vi "ReceiveAsyncMessage.vi"(8 "error in (no error)":errorcluster, 11 "reference input":refnum<k24>) -> (0 "error out":errorcluster, 3 "reference output":refnum<k24>)   [LabVIEW 2013, in "main.lvlib"]
uses:
  main.lvlib
  C:/Users/Simon/SkyDrive/LabView/2013/DM2020/bin/medimatic_bt_receiver.dll
  bin/medimatic_bt_receiver.dll
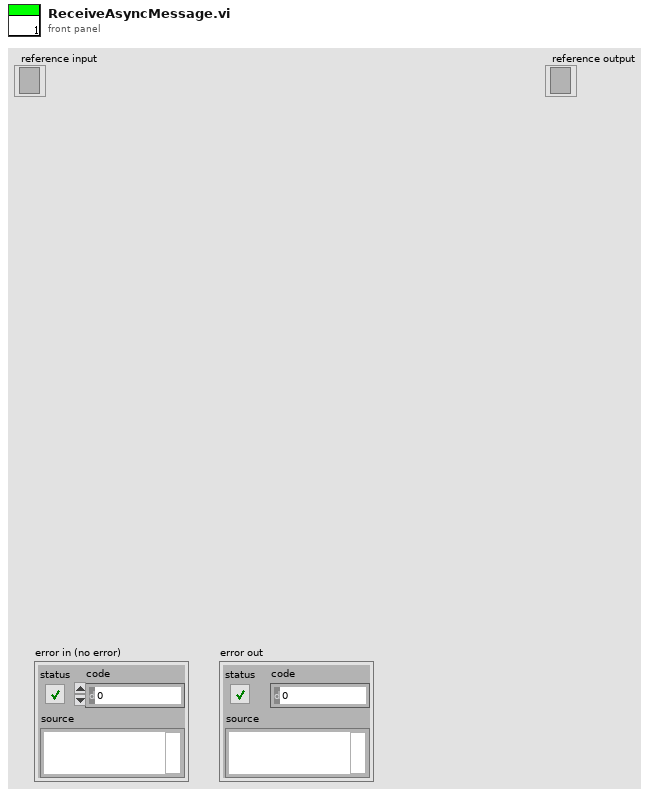
[diagram p1: front panel]
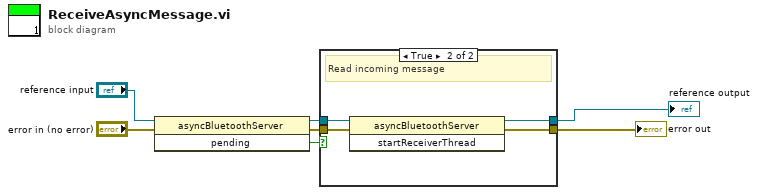
[diagram p0: block diagram]
diagram:
  n1 = invoke class="asyncBluetoothServer" method="pending"(reference="reference input", error in="error in (no error)") -> (reference out=w6:refnum<k24>, error out=w5:errorcluster, "pending"=w7:bool)  [unwired: 1 in]
  n2 = case shown="True" w7 {
    tunnel: [w8 w11] -> w3
    tunnel: [w9 w10] -> w2
    tunnel: w5 -> [w9 w12]
    tunnel: w6 -> [w8 w13]
    frame False {
    }
    frame True {
      # "Read incoming message"
      n3 = invoke class="asyncBluetoothServer" method="startReceiverThread"(reference=w13, error in=w12) -> (reference out=w11:refnum<k24>, error out=w10:errorcluster)  [unwired: 1 in, 1 out]
    }
  }
  "error out" <- w2
  "reference output" <- w3
